vi "to string.vi"(8 "error in":errorcluster, 11 "channel in":refnum<class "fifo channel.lvclass">) -> (0 "error out":errorcluster, 1 "channel data":string, 2 "identifier":string, 3 "channel out":refnum<class "fifo channel.lvclass">)   [LabVIEW 2014, in "fifo channel.lvclass"]
uses:
  fifo channel.lvclass
  fifo channel.lvclass/fifo channel.ctl
  Read fifo config.vi
  <vilib>/NI/Tag Bus Module Framework/channel/TBM channel.lvclass
  <vilib>/NI/Configuration Framework/serializable configuration/NISE_CEF_serializable configuration.lvclass
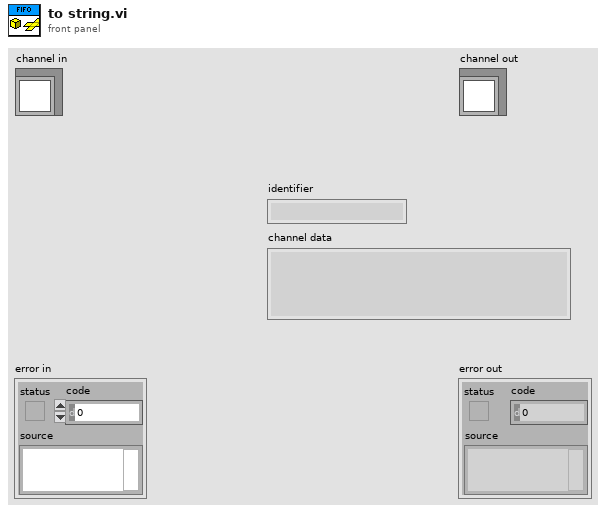
[diagram p1: front panel]
types:
  T1 = typedef "fifo channel.lvclass/fifo channel settings.ctl" = cluster{"Timeout":string, "Reset":string, "Averages":i32, "Samples":u32, "Channels":i32, "Fifo size":u32}
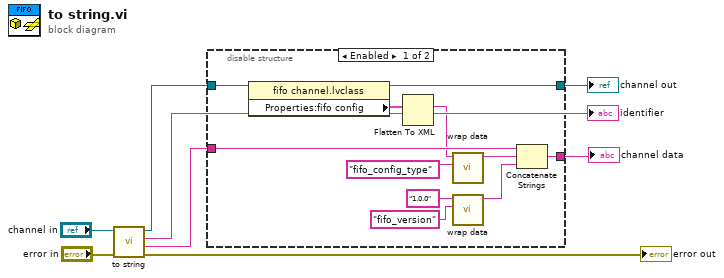
[diagram p0: block diagram]
diagram:
  n1 = call-parent "to string.vi"("error in"="error in", "channel in"="channel in") -> ("error out"=→"error out":errorcluster, "channel data"=w1:string, "identifier"=→"identifier":string, "channel out"=w5:refnum<class "fifo channel.lvclass">)  [unwired: 6 in]
  n2 = disable-structure shown="Enabled" {
    disable-tunnel: w5 -> [w19 w20]
    disable-tunnel: [w18 w20] -> w3
    disable-tunnel: [w13 w21] -> w2
    disable-tunnel: w1 -> [w12 w21]
    frame Enabled {
      n3 = property class="fifo channel.lvclass"(reference=w19) -> (reference out=w18:refnum<class "fifo channel.lvclass">, "Properties:fifo config"=w17:T1)  [unwired: 1 in, 1 out]
      n4 = Flatten To XML(anything=w17) -> (xml string=w10:string)
      n5 = call <vilib>:"wrap data.vi"("identifier"="fifo_config_type" ("additional identifier"), "data to wrap"=w10) -> ("wrapped data"=w11:string)  [unwired: 9 in]
      n6 = call <vilib>:"wrap data.vi"("identifier"="fifo_version", "data to wrap"="1.0.0") -> ("wrapped data"=w9:string)  [unwired: 9 in]
      n7 = Concatenate Strings(w12, w11, w9) -> (w13:string)
    }
    frame Disabled {
    }
  }
  "channel out" <- w3
  "channel data" <- w2
